vi "CRYCheck Open Two Asio Driver.vi"(11 "Selected channel Info":T1[](array[typedef]) {"Coupling" items=["Default"=-1, "RSE"=10083, "NRSE"=10078, "Differential"=10106, "Pseudodifferential"=12529]; "term config" items=["Default"=-1, "RSE"=10083, "NRSE"=10078, "Differential"=10106, "Pseudodifferential"=12529]; "Anti-aliasing Factor (%fs)" format="%.2f"}) -> (3 "Run flag":bool)   [LabVIEW 2013]
uses:
  Typedef Control/CRYHardware Channel Info.ctl
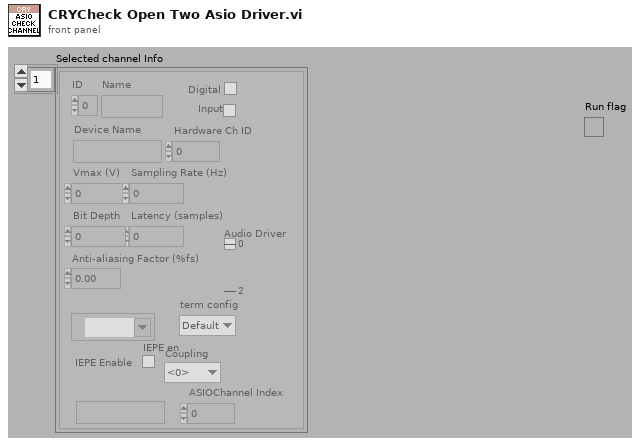
[diagram p1: front panel]
types:
  T1 = typedef "CRYHardware Channel Info.ctl" = cluster{"ID":i32, "Name":string, "Digital":bool, "Input":bool, "Device Name":string, "Hardware Ch ID":u8, "Vmax (V)":dbl, "Latency (samples)":dbl, "Sampling Rate (Hz)":u32, "Bit Depth":u32, "Anti-aliasing Factor (%fs)":sgl, "DAQmx Channel":tag, "term config":i32, "Coupling":i32, "IEPE en":bool, "ASIOChannel Name":string, "Audio Driver":u16, "ASIOChannel Index":u8}
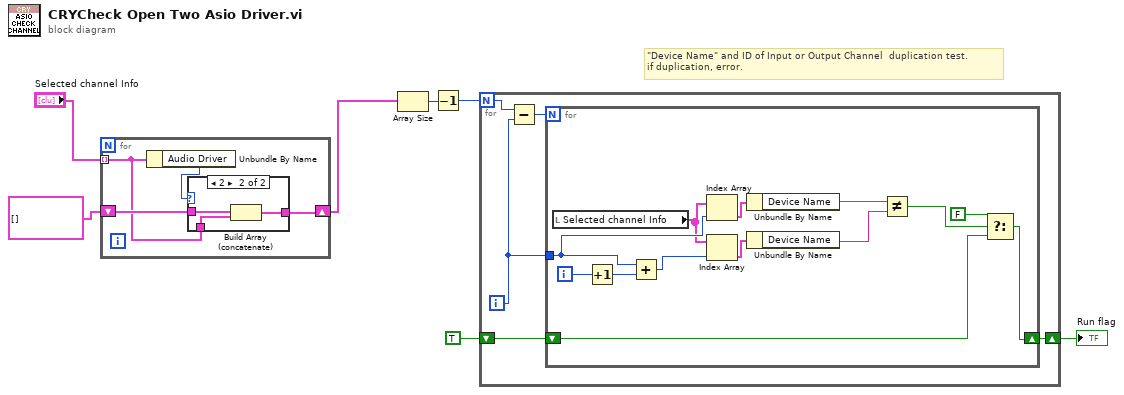
[diagram p0: block diagram]
diagram:
  # "\"Device Name\" and ID of Input or Output Channel  duplication test.\nif duplication, error."
  n1 = for {
    tunnel: "Selected channel Info" -> [w9] mode=indexing
    shift-right: [w8] -> w1
    shift-left: T1[] [] ("Selected channel Info") -> [w10]
    n2 = Unbundle By Name(w9) -> ("Audio Driver"=w11:u16)
    n3 = case shown="2" w11 {
      tunnel: w10 -> [w12 w15]
      tunnel: w9 -> [_ w14]
      tunnel: [w12 w13] -> w8
      frame 0, Default {
      }
      frame 2 {
        n4 = Build Array (concatenate)(w15, w14) -> (w13:T1[])
      }
    }
  }
  n5 = Array Size(array=w1) -> (size(s)=w6:i32)
  n6 = Decrement(x=w6) -> (x-1=w7:i32)
  n7 = for {
    N: w7 -> [w20]
    shift-right: [w17] -> w4
    shift-left: TRUE ("Run flag") -> [w16]
    i -> [w18]
    n8 = Subtract(x=w20, y=w18) -> (x-y=w19:i32)
    n9 = for {
      N: w19 -> [_]
      tunnel: w18 -> [w28]
      shift-right: [w22] -> w17
      shift-left: w16 -> [w23]
      i -> [w31]
      n10 = local read "Selected channel Info"() -> (w27:T1[])
      n11 = Increment(x=w31) -> (x+1=w29:i32)
      n12 = Add(x=w28, y=w29) -> (x+y=w32:i32)
      n13 = Index Array(array=w27, index=w28) -> (element=w30:T1)
      n14 = Index Array(array=w27, index=w32) -> (element=w33:T1)
      n15 = Unbundle By Name(w30) -> ("Device Name"=w25:string)
      n16 = Unbundle By Name(w33) -> ("Device Name"=w26:string)
      n17 = Not Equal?(x=w25, y=w26) -> (x != y?=w21:bool)
      n18 = Select(t=FALSE ("Run flag"), s=w21, f=w23) -> (s? t:f=w22:bool)
    }
  }
  "Run flag" <- w4
